vi "Receive String.vi"(4 "Source (\"\")":string, 6 "Timeout (25000)":u32=25000, 8 "error in (no error)":errorcluster, 11 "VISA resource name":refnum<visa-resource-name>) -> (0 "error out":errorcluster, 1 "Read Buffer":string, 3 "VISA resource name out":refnum<visa-resource-name>)   [LabVIEW 2011, in "Yokogawa DX Series.lvlib"]
doc: "This VI receives a string from the instrument. The terminate of string is CRLF.\nThis returns Read Buffer except CRLF."
uses:
  <instrlib>/Yokogawa DX Series/Yokogawa DX Series.lvlib
panel:
  # "msec"
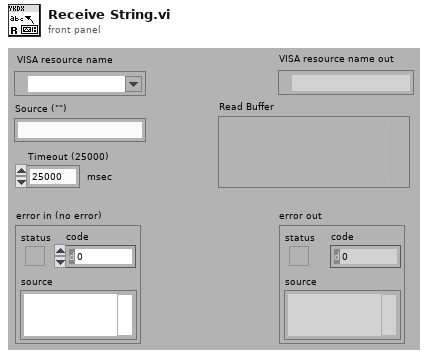
[diagram p1: front panel]
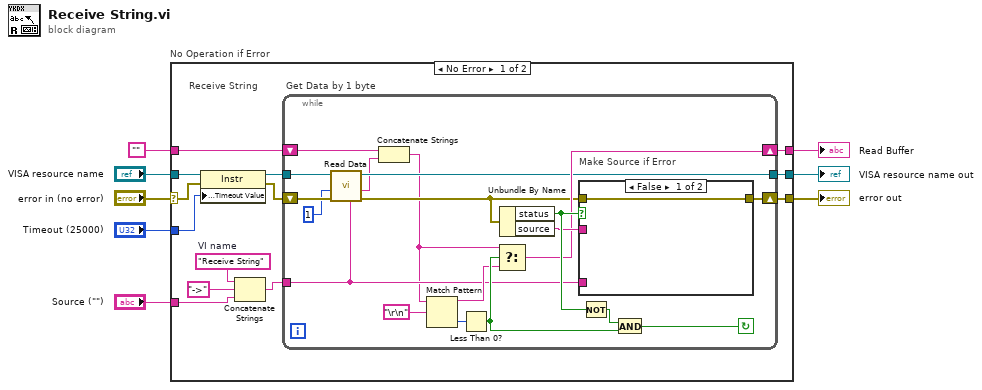
[diagram p0: block diagram]
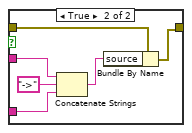
[diagram p2: hidden frame]
diagram:
  n1 = case "No Operation if Error" shown="No Error" "error in (no error)" {
    selector: "error in (no error)" -> [w13 w48]
    tunnel: "VISA resource name" -> [w16 w50]
    tunnel: [w21 w50] -> w5
    tunnel: [w18 w48] -> w8
    tunnel: "Source (\"\")" -> [w9 _]
    tunnel: [w19 w49] -> w6
    tunnel: "" -> [w20 w49]
    tunnel: "Timeout (25000)" -> [w14 _]
    frame No Error {
      w11 = "Receive String"  # VI name
      # "Receive String"
      n2 = property class="Instr"(reference=w16, error in=w13, "General Settings:Timeout Value"=w14) -> (reference out=w15:refnum<visa-resource-name>, error out=w17:errorcluster)
      n3 = Concatenate Strings(w11, "->", w9) -> (w12:string)
      n4 = while "Get Data by 1 byte" {
        shift-left: w17 -> [w29]
        shift-right: [w30] -> w18
        tunnel: w12 -> [w23]
        shift-left: w20 -> [w40]
        shift-right: [w32] -> w19
        tunnel: w15 -> [w24]
        tunnel: [w27] -> w21
        stop <- w37 continue-if-true
        n5 = call <instrlib>:"Read Data.vi"("Source (\"\")"=w23, "error in (no error)"=w29, "Byte (0)"=1, "VISA resource name"=w24) -> ("error out"=w28:errorcluster, "Read Buffer"=w26:string, "VISA resource name out"=w27:refnum<visa-resource-name>)  [unwired: 5 out]
        n6 = Concatenate Strings(w40, w26) -> (w22:string)
        n7 = Match Pattern(string=w22, regular expression="\r\n") -> (before substring=w33:string, offset past match=w38:i32)  [unwired: 3 out]
        n8 = Less Than 0?(x=w38) -> (x < 0?=w34:bool)
        n9 = Select(t=w22, s=w34, f=w33) -> (s? t:f=w32:string)
        n10 = Unbundle By Name(w28) -> ("status"=w36:bool, "source"=w35:string)
        n11 = case "Make Source if Error" shown="False" w36 {
          tunnel: w28 -> [w41 w47]
          tunnel: [w41 w46] -> w30
          tunnel: w35 -> [_ w44]
          tunnel: w23 -> [_ w42]
          frame False {
          }
          frame True {
            n12 = Concatenate Strings(w44, "->", w42) -> (w43:string)
            n13 = Bundle By Name(cluster=w47, "source"=w43) -> (w46:errorcluster)
          }
        }
        n14 = Not(x=w36) -> (.not. x?=w31:bool)
        n15 = And(x=w31, y=w34) -> (x .and. y?=w37:bool)
      }
    }
    frame Error {
    }
  }
  "error out" <- w8
  "VISA resource name out" <- w5
  "Read Buffer" <- w6
